vi "DeactivateChnlHW.vi"(8 "error in (no error)":errorcluster, 11 "BME_DG_Chnl in":refnum<class "BME_DG_Chnl.lvclass">) -> (0 "error out":errorcluster, 3 "BME_DG_Chnl out":refnum<class "BME_DG_Chnl.lvclass">)   [LabVIEW 2009, in "POLARIS BME DG.lvlib" / "BME_DG_Chnl.lvclass"]
doc: "This VI sets the active bit of channel false and calls ModifyChnlHW.vi\n\nATTENTION: direct call of this VI causes asyncronouse HW parameter change. It may be good idea to deactivate some HW before or use synchronus parameter change mechanism in case of SG08P2.\n\n\n---------------\n\nauthor: Alexander Kessler, Helmholtz-Institut-Jena \nmaintainer: Alexander Kessler: alexander.kessler@uni-jena.de\n\n\nLicense Agreement for this software:\n\nCopyright (C)\nHelmholtz-Institut-Jena\nFröbelsteg 3\n07743 Jena\nGermany\n\nContact: alexander.kessler@uni-jena.de\n\nThis program is free software; you can redistribute it and/or modify it under the terms of the GNU General Public License as published by the Free Software Foundation; either version 2 of the license, or (at your option) any later version.\n\nThis program is distributed in the hope that it will be useful, but WITHOUT ANY WARRANTY; without even the implied warranty of MERCHANTABILITY or FITNESS FOR A PARTICULAR PURPOSE. See the GNU General License for more details (http://www.gnu.org)."
uses:
  BME_DG_Chnl.lvclass
  BME_DG_Chnl.lvclass/BME_DG_Chnl.ctl
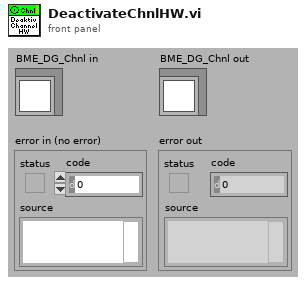
[diagram p1: front panel]
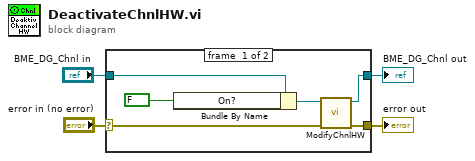
[diagram p0: block diagram]
diagram:
  n1 = case shown="No Error" "error in (no error)" {
    selector: "error in (no error)" -> [w6 w12]
    tunnel: [w5 w12] -> w3
    tunnel: [w7 w11] -> w1
    tunnel: "BME_DG_Chnl in" -> [w10 w11]
    frame #0 {
      n2 = Bundle By Name(cluster=w10, "On?"=FALSE ("ChnParameter.On? (false)")) -> (w8:refnum<class "BME_DG_Chnl.lvclass">)
      n3 = call-dynamic "ModifyChnlHW.vi"("error in (no error)"=w6, "BME_DG_Chnl in"=w8) -> ("error out"=w5:errorcluster, "BME_DG_Chnl out"=w7:refnum<class "BME_DG_Chnl.lvclass">)  [unwired: 8 in]
    }
    frame #1 {
    }
  }
  "error out" <- w3
  "BME_DG_Chnl out" <- w1
